vi "LightControl.vi"(8 "Light overide off":bool, 11 "Light":bool) -> (3 "RelayValue":T1)   [LabVIEW 2016]
uses:
  <vilib>/Rock Robotics/WPI/Relay/WPI_RelayValue.ctl
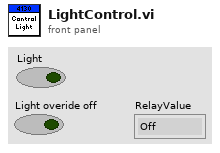
[diagram p1: front panel]
types:
  T1 = typedef "WPI_RelayValue.ctl" = enum16{"Off", "On", "Forward", "Reverse"}
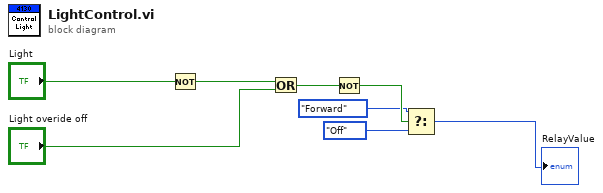
[diagram p0: block diagram]
diagram:
  n1 = Not(x="Light") -> (.not. x?=w5:bool)
  n2 = Or(x=w5, y="Light overide off") -> (x .or. y?=w7:bool)
  n3 = Not(x=w7) -> (.not. x?=w8:bool)
  n4 = Select(t=WPI_RelayValue."Forward" ("RelayValue"), s=w8, f=WPI_RelayValue."Off" ("RelayValue")) -> (s? t:f=→"RelayValue":T1)
